vi "Camera_Trigger_Manual.vi"() -> ()   [LabVIEW 2022 SP3]
panel:
  in  "Trigger State":bool
  out "Cam 2":bool
  out "Cam 1":bool
  # "HW Trigger Control"
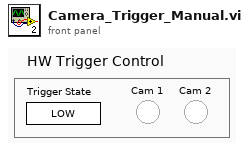
[diagram p1: front panel]
types:
  T1 = enum32{"Invalid", "Standard", "Closed", "Hidden", "Minimized", "Maximized"}
  T2 = enum32{"invalid app kind", "Development System", "Run Time System", "Student Edition", "Embedded LabVIEW", "Evaluation", "Custom"}
  T3 = typedef "Data.ctl" = cluster{"system":cluster{"info":cluster{"menuSelect":u16, "version":u16, "serial":string, "captureActive":bool, "captureBegin":bool, "emptyAndRefill":bool}, "userInfo":cluster{"operatorName":string, "date":timestamp}, "camera":cluster{"exposureTime":i32, "aperture":enum32{"Item 0", "Item 1", "Item 2", "Item 3"}, "framerate":i32, "framerateMax":i32, "legacyAttributes":bool}}, "connections":cluster{"arduino":cluster{"connection":refnum<visa-resource-name>, "status":bool, "openState":bool, "emptyStart":u32}, "pump":cluster{"connection":refnum<visa-resource-name>, "status":bool, "command":string, "dispenseSpeed":i32, "flushSize":i32}, "camera":cluster{"cam1":cluster{"connection":T4, "status":bool}, "cam2":cluster{"connection":T4, "status":bool}}}, "queue":cluster{"process":cluster{"cam1":refnum<queue>, "cam2":refnum<queue>, "queueSize":i32}, "save":cluster{"cam1":refnum<queue>, "cam2":refnum<queue>, "queueSize":i32}, "overloadThreshold":i32}, "imageProcess":cluster{"cam1":cluster{"preAllocation":cluster{"image":T5, "originalDisplay":T5, "originalRgb":T5, "binary":T5, "save":T5, "calibrationFull":T5, "calibrationDetect":T5}, "calibration":cluster{"pathFull":path, "pathDetect":path, "ROI":T6}}, "cam2":cluster{"preAllocation":cluster{"image":T5, "originalDisplay":T5, "originalRgb":T5, "binary":T5, "save":T5, "calibrationFull":T5, "calibrationDetect":T5}, "calibration":cluster{"pathFull":path, "pathDetect":path, "ROI":T6}}, "process":cluster{"planeExtract":T5, "planeSubtract":T5, "cropMask":T5}, "detection":cluster{"sampleTimeout":i32, "sizeThreshold":i32, "detectionRegionPct":dbl}}, "sampleData":cluster{"sampleId":string, "projectId":string, "voucherID":string, "speciesName":string, "collectionDate":timestamp, "sampleStation":string, "location":string, "lat":dbl, "lon":dbl, "determiner":string, "sex":string, "otherNotes":string}, "Session In":T4}
  T4 = typedef "IMAQdx.ctl" = refnum<k21>
  T5 = typedef "IMAQ Image.ctl" = refnum<image>
  T6 = typedef "IMAQ Rectangle" = cluster{"Left":i32, "Top":i32, "Right":i32, "Bottom":i32, "Rotation":dbl}
  T7 = cluster{"Core":cluster{"Current VI Reference":refnum<vi>, "Close Panel on Exit?":bool}, "value":T3}
  T8 = cluster{"Current VI Reference":refnum<vi>, "Close Panel on Exit?":bool}
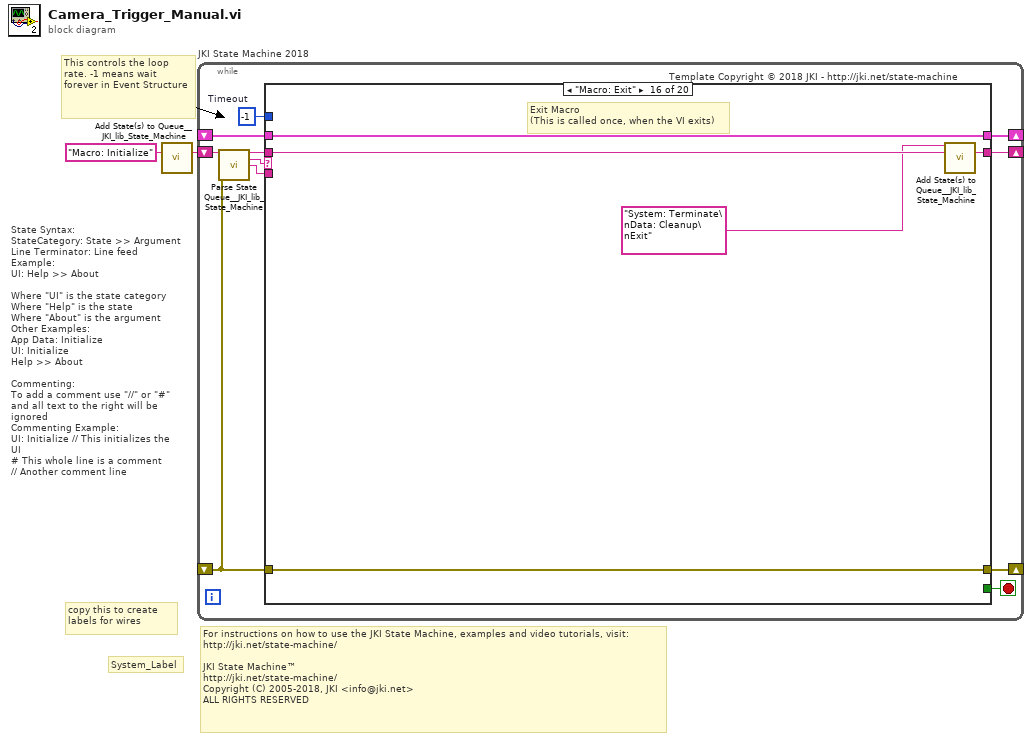
[diagram p0: block diagram]
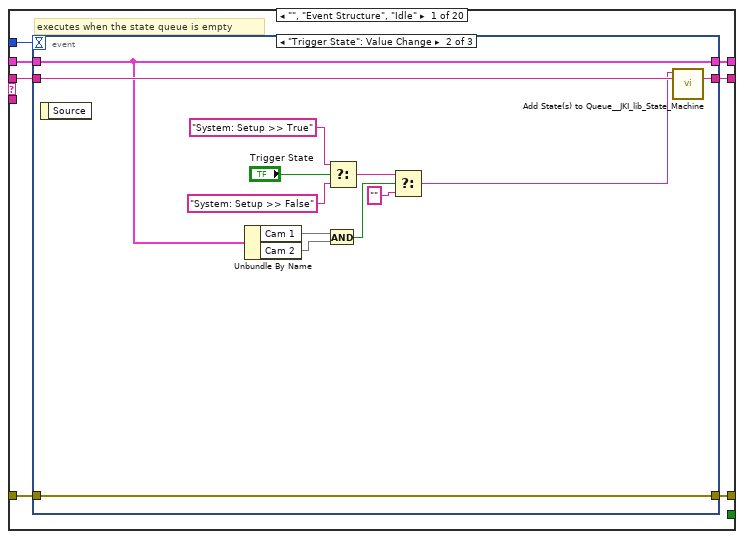
[diagram p2: hidden frame]
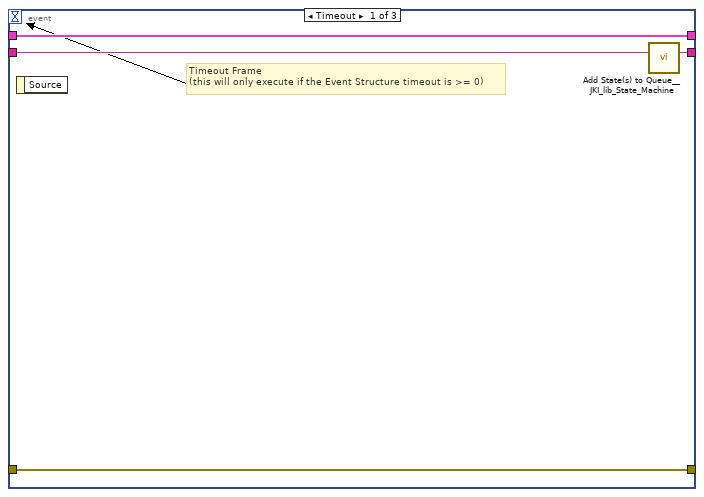
[diagram p3: hidden frame]
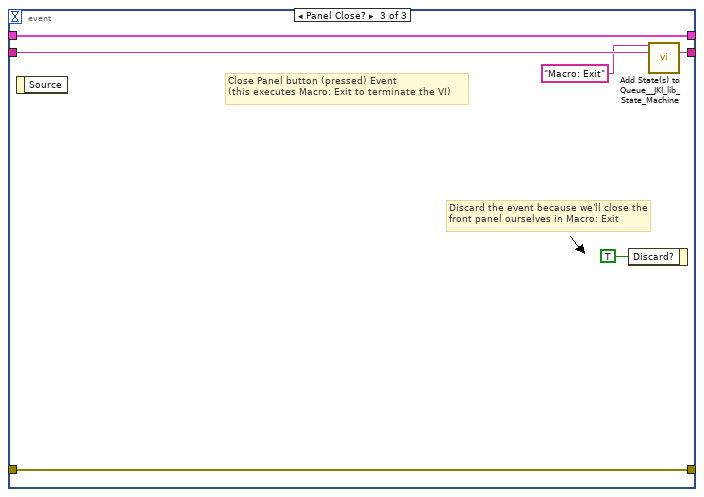
[diagram p4: hidden frame]
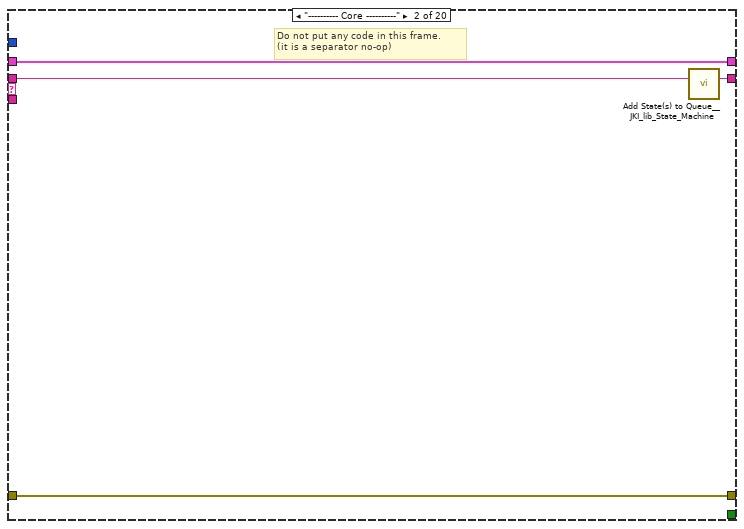
[diagram p5: hidden frame]
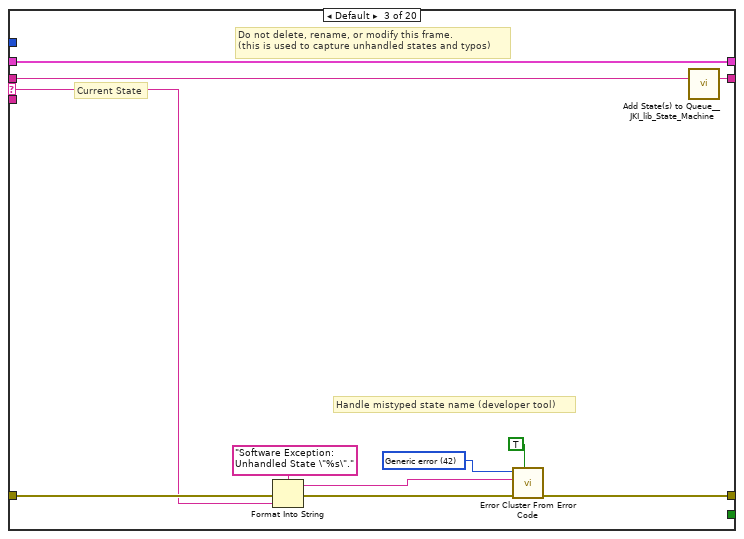
[diagram p6: hidden frame]
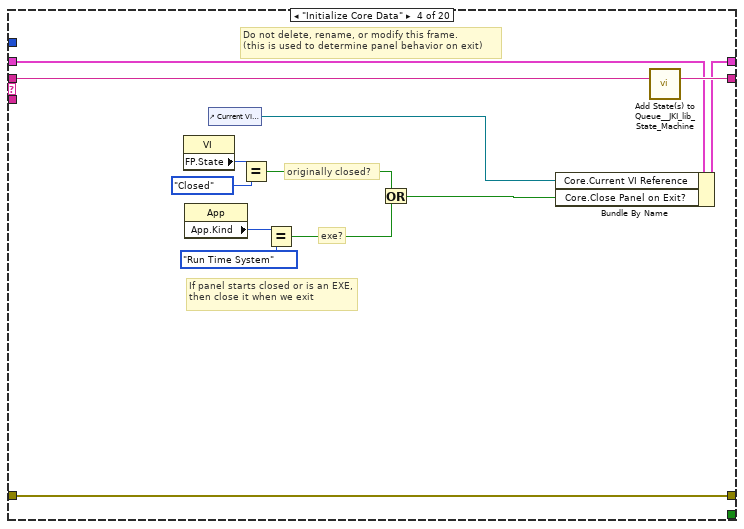
[diagram p7: hidden frame]
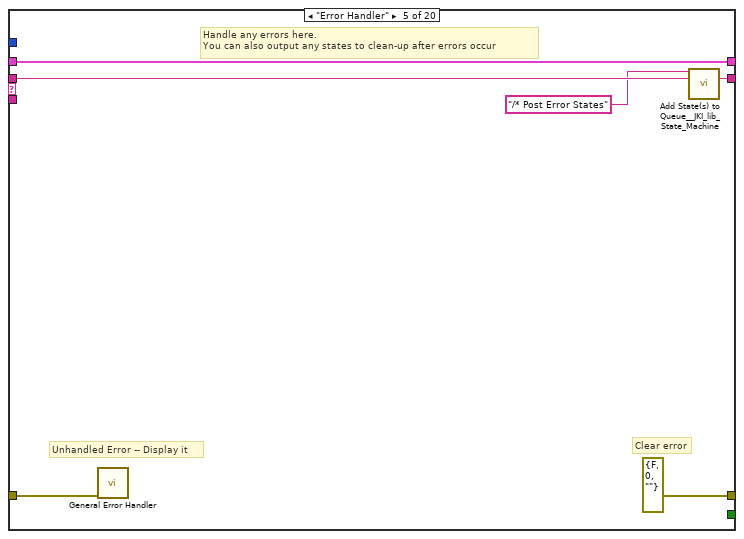
[diagram p8: hidden frame]
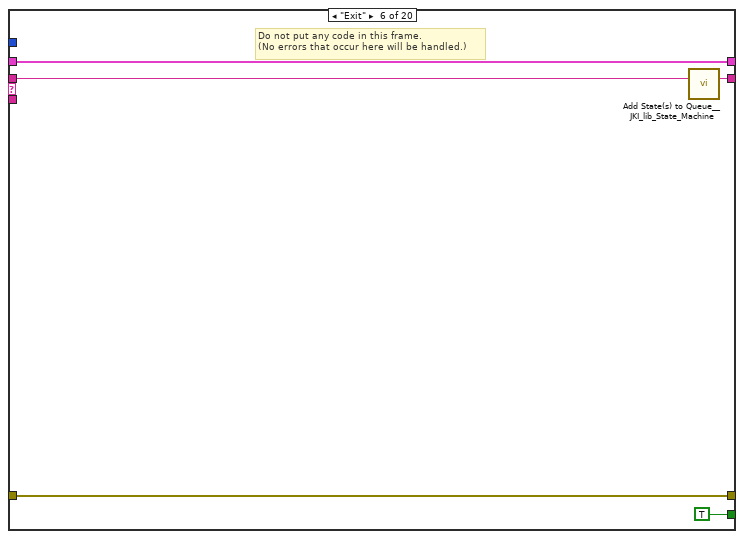
[diagram p9: hidden frame]
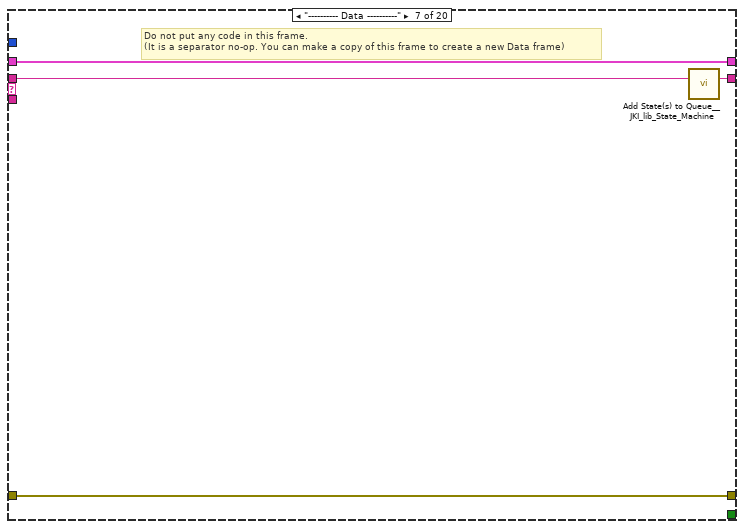
[diagram p10: hidden frame]
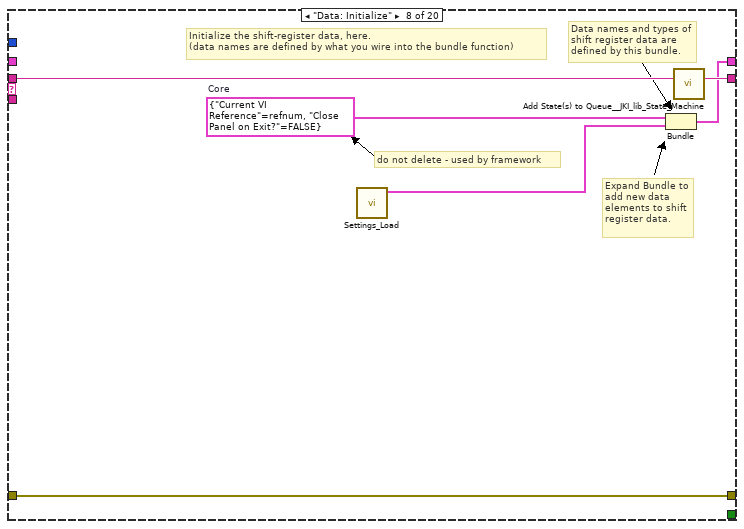
[diagram p11: hidden frame]
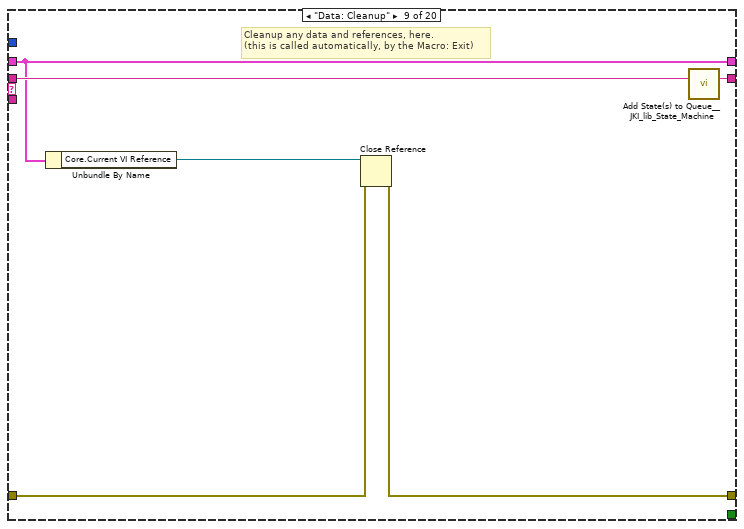
[diagram p12: hidden frame]
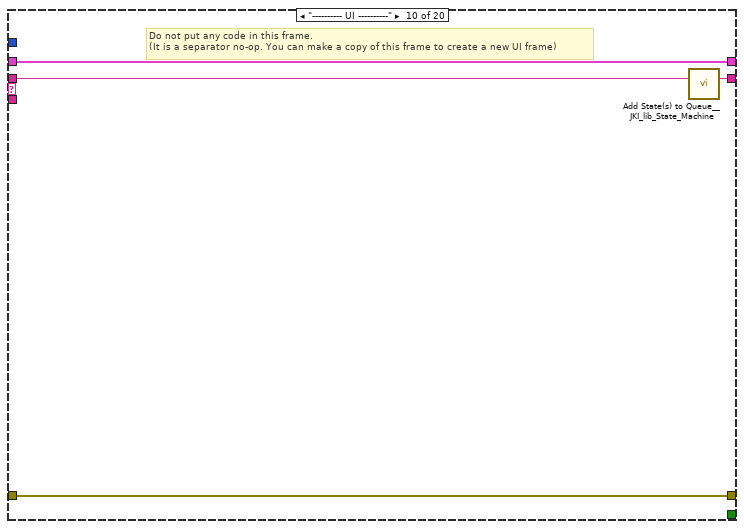
[diagram p13: hidden frame]
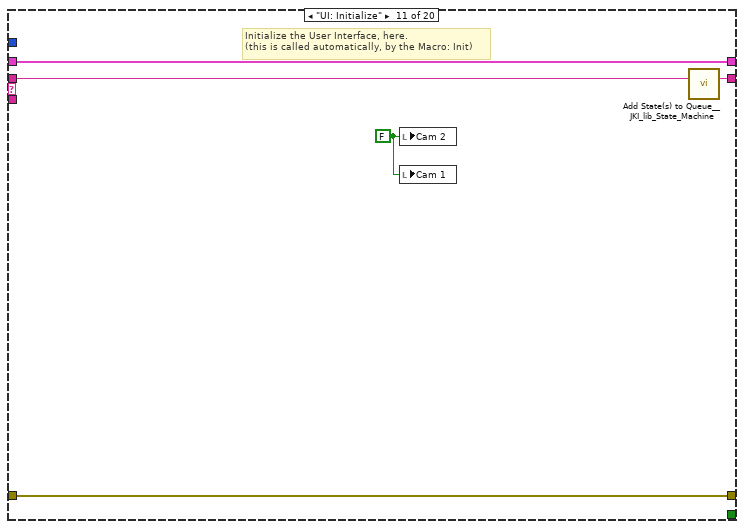
[diagram p14: hidden frame]
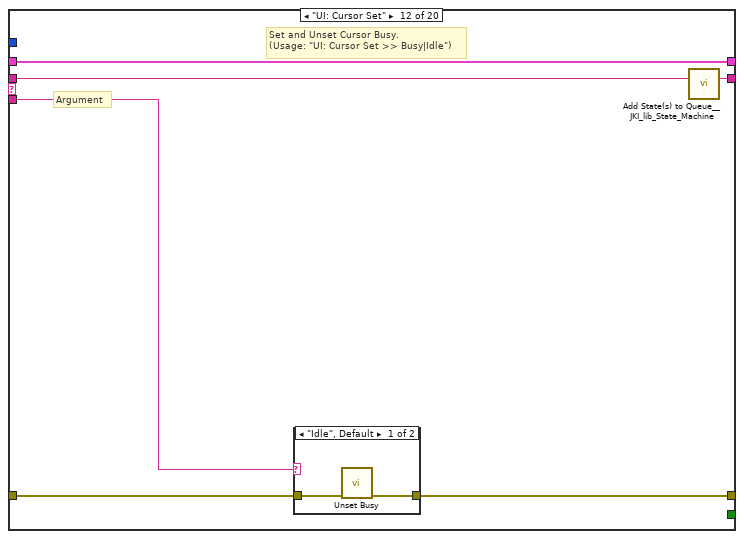
[diagram p15: hidden frame]
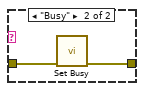
[diagram p16: hidden frame]
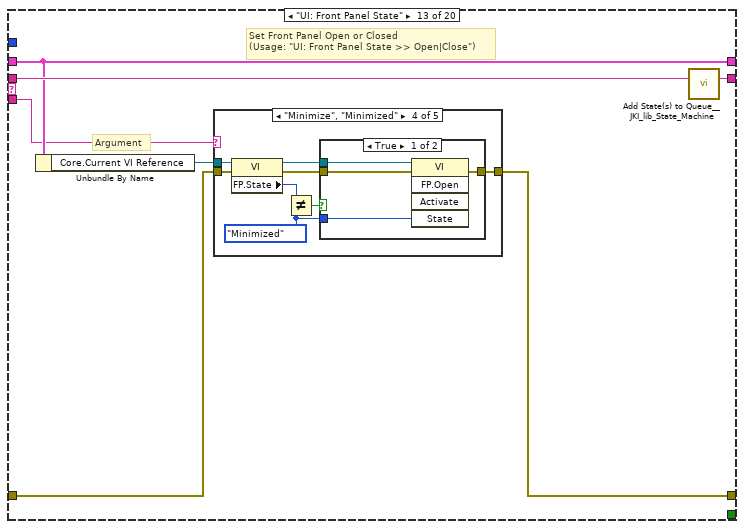
[diagram p17: hidden frame]
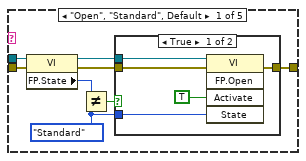
[diagram p18: hidden frame]
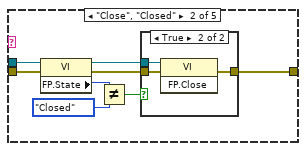
[diagram p20: hidden frame]
diagram:
  # "For instructions on how to use the JKI State Machine, examples and video tutorials, visit:\nhttp://jki.net/state-machine/\n\nJKI State Machine™\nhttp://jki.net/state-machine/\nCopyright (C) 2005-2018, JKI <info@jki.net>\nALL RIGHTS RESERVED"
  # "State Syntax:\nStateCategory: State >> Argument\nLine Terminator: Line feed\nExample:\nUI: Help >> About\n\nWhere \"UI\" is the state category\nWhere \"Help\" is the state\nWhere \"About\" is the argument\nOther Examples:\nApp Data: Initialize\nUI: Initialize\nHelp >> About\n\nCommenting:\nTo add a comment use \"//\" or \"#\" and all text to the right will be ignored\nCommenting Example:\nUI: Initialize // This initializes the UI\n# This whole line is a comment\n// Another comment line"
  # "copy this to create labels for wires"
  # "This controls the loop rate. -1 means wait forever in Event Structure"
  # "System_Label"
  n1 = call <vilib>:"Add State(s) to Queue__JKI_lib_State_Machine.vi"("State(s) in (\"\")"="Macro: Initialize") -> ("States Out"=w2:string)  [unwired: 14 in]
  n2 = while "JKI State Machine 2018" {
    shift-right: [w6] -> _
    shift-left: _ -> [w5]
    shift-right: [w9] -> _
    shift-left: _ -> [w3]
    shift-right: [w8] -> _
    shift-left: w2 -> [w10]
    stop <- w7 stop-if-true
    w4 = -1  # Timeout
    # "Template Copyright © 2018 JKI - http://jki.net/state-machine"
    n3 = call <vilib>:"Parse State Queue__JKI_lib_State_Machine.vi"("State Queue"=w10, "Error In (no error)"=w3) -> ("Remaining States"=w12:string, "Current State"=w13:string, "Arguments"=w11:string)  [unwired: 11 in]
    n4 = case shown="\"Macro: Exit\"" w13 {
      selector: w13 -> [_ _ w48 _ _ _ _ _ _ _ _ _ _ _ _ _ _ _ _ _]
      tunnel: w12 -> [w20 w47 w52 w71 w77 w82 w86 w92 w98 w102 w107 w113 w124 w193 w198 w203 w207 w218 w225 w233]
      tunnel: w11 -> [_ _ _ _ _ _ _ _ _ _ _ w108 w118 _ _ _ _ _ _ w228]
      tunnel: w5 -> [w18 w44 w50 w64 w74 w80 w83 _ w93 w99 w105 w111 w120 w190 w195 w200 w204 w213 w221 w231]
      tunnel: [w17 w45 w54 w68 errorcluster {"status"=FALSE, "code"=0, "source"=""} ("error out") w79 w84 w89 w94 w100 w104 w109 w121 w191 w196 w201 w205 w216 w223 w226] -> w9
      tunnel: w3 -> [w16 w45 w53 w68 w73 w79 w84 w89 w95 w100 w104 w110 w122 w191 w196 w201 w205 w216 w223 w230]
      tunnel: [w19 w46 w51 w70 w76 w81 w85 w91 w97 w101 w106 w112 w123 w192 w197 w202 w206 w217 w224 w232] -> w8
      tunnel: [_ _ _ _ _ TRUE _ _ _ _ _ _ _ _ _ _ _ _ _ _] -> w7
      tunnel: [w15 w44 w50 w69 w74 w80 w83 w90 w93 w99 w105 w111 w120 w190 w195 w200 w204 w211 w220 w231] -> w6
      tunnel: w4 -> [w14 _ _ _ _ _ _ _ _ _ _ _ _ _ _ _ _ _ _ _]
      frame "", "Event Structure", "Idle" {
        # "executes when the state queue is empty"
        n5 = event shown="[1] \"Trigger State\": Value Change" {
          selector: _ -> [_ _ _]
          dyn-events: _ -> [_ _ _]
          timeout: w14 -> [_ _ _]
          tunnel: w20 -> [w24 w37 w43]
          tunnel: [w23 w36 w42] -> w19
          tunnel: w18 -> [w21 w32 w40]
          tunnel: [w22 w35 w41] -> w17
          tunnel: w16 -> [w22 w35 w41]
          tunnel: [w21 w32 w40] -> w15
          event Timeout {
            # "Timeout Frame\n(this will only execute if the Event Structure timeout is >= 0)"
            n6 = event-data() -> ()  [unwired: 1 in, 1 out]
            n7 = call <vilib>:"Add State(s) to Queue__JKI_lib_State_Machine.vi"("State(s) in (\"\")"=w24) -> ("States Out"=w23:string)  [unwired: 14 in]
          }
          event "Trigger State": Value Change {
            n8 = event-data() -> ()  [unwired: 1 in, 1 out]
            n9 = Unbundle By Name(w32) -> ("Cam 1"=w30, "Cam 2"=w29)
            n10 = And(x=w30, y=w29) -> (x .and. y?=w28:bool)
            n11 = Select(t="System: Setup >> True" ("State(s) in Front (\"\")"), s="Trigger State", f="System: Setup >> False" ("State(s) in Front (\"\")")) -> (s? t:f=w27:string)
            n12 = Select(t=w27, s=w28, f="") -> (s? t:f=w25:string)
            n13 = call <vilib>:"Add State(s) to Queue__JKI_lib_State_Machine.vi"("State(s) in Front (\"\")"=w25, "State(s) in (\"\")"=w37) -> ("States Out"=w36:string)  [unwired: 13 in]
          }
          event Panel Close? {
            # "Discard the event because we'll close the front panel ourselves in Macro: Exit"
            # "Close Panel button (pressed) Event\n(this executes Macro: Exit to terminate the VI)"
            n14 = event-data() -> ()  [unwired: 1 in, 1 out]
            n15 = event-data("Discard?"=TRUE) -> ()  [unwired: 1 in, 1 out]
            n16 = call <vilib>:"Add State(s) to Queue__JKI_lib_State_Machine.vi"("State(s) in Front (\"\")"="Macro: Exit", "State(s) in (\"\")"=w43) -> ("States Out"=w42:string)  [unwired: 13 in]
          }
        }
      }
      frame "---------- Core ----------" {
        # "Do not put any code in this frame.\n(it is a separator no-op)"
        n17 = call <vilib>:"Add State(s) to Queue__JKI_lib_State_Machine.vi"("State(s) in (\"\")"=w47) -> ("States Out"=w46:string)  [unwired: 14 in]
      }
      frame Default {
        w57 = 42 items=["No error", "Argument error", "Memory is full", "Out of zone", "End of file", "File already open", "Generic file I/O error", "File not found", "File permission error", "Disk is full", "Duplicate path", "Too many files open", "System feature not enabled", "Resource file not found", "Cannot add resource", "Resource not found", "Image not found", "Image memory error", "Pen does not exist", "Config type invalid", "Config token not found", "Config parse error", "Config memory error", "Bad external code format", "Bad external code offset", "External code not present", "Null window", "Destroy window error", "Null menu", "Print aborted", "Bad print record", "Print driver error", "Windows error during printing", "Memory error during printing", "Print dialog error", "Generic print error", "Invalid device refnum", "Device not found", "Device parameter error", "Device unit error", "Cannot open device", "Device call aborted", "Generic error", "Cancelled by user", "Object ID too low", "Object ID too high", "Object not in heap", "Unknown heap", "Unknown object (invalid DefProc)", "Unknown object (DefProc not in table)", "Message out of range", "Invalid (null) method", "Unknown message", "Manager call not supported", "Bad address", "Network operation in progress", "Network operation timed out", "Connection is busy", "Network attribute not supported", "Network error", "Address in use", "System out of memory", "Connection aborted", "Connection refused", "Not connected", "Already connected", "Connection closed", "Initialization error (interapplication manager)", "Bad occurrence", "Wait on unbound occurrence handler", "Occurrence queue overflow", "Datalog type conflict", "Unused", "Unrecognized type (interapplication manager)", "Memory corrupt", "Failed to make temporary DLL", "Old CIN version", "Drag socket not found", "Failed to load drop-object", "Failed to register OLE object", "Failed to release OLE object", "Format specifier type mismatch", "Unknown format specifier", "Too few format specifiers", "Too many format specifiers", "Scan failed", "Newer CIN version", "Error converting to variant", "Runtime menu error", "Password tampered", "Variant attribute not found", "Incompatible variant data type", "Event data is not available", "Event Store is not present", "Occurrence is not found", "Event Queue is not created", "Event info is not available", "Refnum passed is NULL", "Error retrieving Class GUID", "Error retrieving CoClass GUID", "Error retrieving TypeLib GUID.", "Bad built application magic bytes.", "Specific driver is different from the specific driver associated with the Logical Name.", "There is no session opened to the class driver.", "Max Error", "MAX - Error with config objects", "MAX - Error loading configuration", "MAX - Group not supported"]
        # "Current State"
        # "Do not delete, rename, or modify this frame.\n(this is used to capture unhandled states and typos)"
        # "Handle mistyped state name (developer tool)"
        n18 = Format Into String(format string="Software Exception: Unhandled State \"%s\"." ("message"), error in=w53, w48) -> (resulting string=w56:string, error out=w55:errorcluster)  [unwired: 1 in]
        n19 = call <vilib>:"Error Cluster From Error Code.vi"("show call chain? (False)"=TRUE, "error in (no error)"=w55, "error message (\"\")"=w56, "error code (0)"=w57) -> ("error out"=w54:errorcluster)  [unwired: 5 in]
        n20 = call <vilib>:"Add State(s) to Queue__JKI_lib_State_Machine.vi"("State(s) in (\"\")"=w52) -> ("States Out"=w51:string)  [unwired: 14 in]
      }
      frame "Initialize Core Data" {
        # "Do not delete, rename, or modify this frame.\n(this is used to determine panel behavior on exit)"
        # "originally closed?"
        # "exe?"
        # "If panel starts closed or is an EXE, then close it when we exit"
        n21 = property class="VI"() -> ("FP.State"=w61:T1)  [unwired: 2 in, 2 out]
        n22 = property class="App"() -> ("App.Kind"=w67:T2)  [unwired: 2 in, 2 out]
        n23 = control-ref of="Current VI Reference"() -> (w62:refnum<vi>)
        n24 = Equal?(x=w61, y=T1."Closed" ("Front Panel Window:State")) -> (x = y?=w59:bool)
        n25 = Equal?(x=w67, y=T2."Run Time System" ("Application:Kind")) -> (x = y?=w65:bool)
        n26 = Or(x=w59, y=w65) -> (x .or. y?=w63:bool)
        n27 = Bundle By Name(cluster=w64, "Core.Current VI Reference"=w62, "Core.Close Panel on Exit?"=w63) -> (w69:T7)
        n28 = call <vilib>:"Add State(s) to Queue__JKI_lib_State_Machine.vi"("State(s) in (\"\")"=w71) -> ("States Out"=w70:string)  [unwired: 14 in]
      }
      frame "Error Handler" {
        # "Unhandled Error -- Display it"
        # "Handle any errors here.\nYou can also output any states to clean-up after errors occur"
        # "Clear error"
        n29 = call <vilib>:"General Error Handler.vi"("error in (no error)"=w73) -> ()  [unwired: 10 in, 5 out]
        n30 = call <vilib>:"Add State(s) to Queue__JKI_lib_State_Machine.vi"("State(s) in Front (\"\")"="/* Post Error States", "State(s) in (\"\")"=w77) -> ("States Out"=w76:string)  [unwired: 13 in]
      }
      frame "Exit" {
        # "Do not put any code in this frame.\n(No errors that occur here will be handled.)"
        n31 = call <vilib>:"Add State(s) to Queue__JKI_lib_State_Machine.vi"("State(s) in (\"\")"=w82) -> ("States Out"=w81:string)  [unwired: 14 in]
      }
      frame "---------- Data ----------" {
        # "Do not put any code in this frame.\n(It is a separator no-op. You can make a copy of this frame to create a new Data frame)"
        n32 = call <vilib>:"Add State(s) to Queue__JKI_lib_State_Machine.vi"("State(s) in (\"\")"=w86) -> ("States Out"=w85:string)  [unwired: 14 in]
      }
      frame "Data: Initialize" {
        w88 = T8 {"Current VI Reference"=refnum, "Close Panel on Exit?"=FALSE}  # Core
        # "do not delete - used by framework"
        # "Expand Bundle to add new data elements to shift register data."
        # "Data names and types of shift register data are defined by this bundle."
        # "Initialize the shift-register data, here.\n(data names are defined by what you wire into the bundle function)"
        n33 = call "Settings_Load.vi"() -> ("value"=w87:T3)  [unwired: 10 in, 1 out]
        n34 = Bundle("Core"=w88, "value"=w87) -> (w90:T7)  [unwired: 1 in]
        n35 = call <vilib>:"Add State(s) to Queue__JKI_lib_State_Machine.vi"("State(s) in (\"\")"=w92) -> ("States Out"=w91:string)  [unwired: 14 in]
      }
      frame "Data: Cleanup" {
        # "Cleanup any data and references, here.\n(this is called automatically, by the Macro: Exit)"
        n36 = Unbundle By Name(w93) -> ("Core.Current VI Reference"=w96:refnum<vi>)
        n37 = Close Reference(reference=w96, error in (no error)=w95) -> (error out=w94:errorcluster)
        n38 = call <vilib>:"Add State(s) to Queue__JKI_lib_State_Machine.vi"("State(s) in (\"\")"=w98) -> ("States Out"=w97:string)  [unwired: 14 in]
      }
      frame "---------- UI ----------" {
        # "Do not put any code in this frame.\n(It is a separator no-op. You can make a copy of this frame to create a new UI frame)"
        n39 = call <vilib>:"Add State(s) to Queue__JKI_lib_State_Machine.vi"("State(s) in (\"\")"=w102) -> ("States Out"=w101:string)  [unwired: 14 in]
      }
      frame "UI: Initialize" {
        w103 = FALSE ("Cam 2")
        # "Initialize the User Interface, here.\n(this is called automatically, by the Macro: Init)"
        n40 = local write "Cam 2"(w103) -> ()
        n41 = local write "Cam 1"(w103) -> ()
        n42 = call <vilib>:"Add State(s) to Queue__JKI_lib_State_Machine.vi"("State(s) in (\"\")"=w107) -> ("States Out"=w106:string)  [unwired: 14 in]
      }
      frame "UI: Cursor Set" {
        # "Argument"
        # "Set and Unset Cursor Busy.\n(Usage: \"UI: Cursor Set >> Busy|Idle\")"
        n43 = case shown="\"Idle\", Default" w108 {
          tunnel: w110 -> [w115 w117]
          tunnel: [w114 w116] -> w109
          frame "Idle", Default {
            n44 = call <vilib>:"Unset Busy.vi"("error in (no error)"=w115) -> ("error out"=w114:errorcluster)  [unwired: 10 in]
          }
          frame "Busy" {
            n45 = call <vilib>:"Set Busy.vi"("error in (no error)"=w117) -> ("error out"=w116:errorcluster)  [unwired: 9 in, 1 out]
          }
        }
        n46 = call <vilib>:"Add State(s) to Queue__JKI_lib_State_Machine.vi"("State(s) in (\"\")"=w113) -> ("States Out"=w112:string)  [unwired: 14 in]
      }
      frame "UI: Front Panel State" {
        # "Argument"
        # "Set Front Panel Open or Closed\n(Usage: \"UI: Front Panel State >> Open|Close\")"
        n47 = Unbundle By Name(w120) -> ("Core.Current VI Reference"=w119:refnum<vi>)
        n48 = case shown="\"Minimize\", \"Minimized\"" w118 {
          tunnel: w122 -> [w130 w145 w156 w169 w182]
          tunnel: [w132 w146 w158 w171 w184] -> w121
          tunnel: w119 -> [w131 w143 w157 w170 w183]
          frame "Open", "Standard", Default {
            w125 = T1."Standard" ("State")
            n49 = property class="VI"(reference=w131, error in=w130) -> (reference out=w128:refnum<vi>, error out=w129:errorcluster, "FP.State"=w127:T1)
            n50 = Not Equal?(x=w127, y=w125) -> (x != y?=w126:bool)
            n51 = case shown="True" w126 {
              tunnel: [w136 w138] -> w132
              tunnel: w129 -> [w135 w138]
              tunnel: w128 -> [w134 _]
              tunnel: w125 -> [w133 _]
              frame True {
                n52 = invoke class="VI" method="FP.Open"(reference=w134, error in=w135, "Activate"=TRUE, "State"=w133) -> (error out=w136:errorcluster)  [unwired: 1 in, 4 out]
              }
              frame False {
              }
            }
          }
          frame "Close", "Closed" {
            n53 = property class="VI"(reference=w143, error in=w145) -> (reference out=w142:refnum<vi>, error out=w144:errorcluster, "FP.State"=w140:T1)
            n54 = Not Equal?(x=w140, y=T1."Closed" ("Front Panel Window:State")) -> (x != y?=w139:bool)
            n55 = case shown="True" w139 {
              tunnel: [w147 w150] -> w146
              tunnel: w144 -> [w147 w149]
              tunnel: w142 -> [_ w148]
              frame False {
              }
              frame True {
                n56 = invoke class="VI" method="FP.Close"(reference=w148, error in=w149) -> (error out=w150:errorcluster)  [unwired: 1 in, 2 out]
              }
            }
          }
          frame "Hidden", "Hide" {
            w151 = T1."Hidden" ("State")
            n57 = property class="VI"(reference=w157, error in=w156) -> (reference out=w154:refnum<vi>, error out=w155:errorcluster, "FP.State"=w153:T1)
            n58 = Not Equal?(x=w153, y=w151) -> (x != y?=w152:bool)
            n59 = case shown="True" w152 {
              tunnel: [w162 w163] -> w158
              tunnel: w155 -> [w161 w163]
              tunnel: w154 -> [w160 _]
              tunnel: w151 -> [w159 _]
              frame True {
                n60 = invoke class="VI" method="FP.Open"(reference=w160, error in=w161, "State"=w159) -> (error out=w162:errorcluster)  [unwired: 2 in, 4 out]
              }
              frame False {
              }
            }
          }
          frame "Minimize", "Minimized" {
            w164 = T1."Minimized" ("State")
            n61 = property class="VI"(reference=w170, error in=w169) -> (reference out=w167:refnum<vi>, error out=w168:errorcluster, "FP.State"=w166:T1)
            n62 = Not Equal?(x=w166, y=w164) -> (x != y?=w165:bool)
            n63 = case shown="True" w165 {
              tunnel: [w175 w176] -> w171
              tunnel: w168 -> [w174 w176]
              tunnel: w167 -> [w173 _]
              tunnel: w164 -> [w172 _]
              frame True {
                n64 = invoke class="VI" method="FP.Open"(reference=w173, error in=w174, "State"=w172) -> (error out=w175:errorcluster)  [unwired: 2 in, 4 out]
              }
              frame False {
              }
            }
          }
          frame "Maximize", "Maximized" {
            w177 = T1."Maximized" ("State")
            n65 = property class="VI"(reference=w183, error in=w182) -> (reference out=w180:refnum<vi>, error out=w181:errorcluster, "FP.State"=w179:T1)
            n66 = Not Equal?(x=w179, y=w177) -> (x != y?=w178:bool)
            n67 = case shown="True" w178 {
              tunnel: [w188 w189] -> w184
              tunnel: w181 -> [w187 w189]
              tunnel: w180 -> [w186 _]
              tunnel: w177 -> [w185 _]
              frame True {
                n68 = invoke class="VI" method="FP.Open"(reference=w186, error in=w187, "State"=w185) -> (error out=w188:errorcluster)  [unwired: 2 in, 4 out]
              }
              frame False {
              }
            }
          }
        }
        n69 = call <vilib>:"Add State(s) to Queue__JKI_lib_State_Machine.vi"("State(s) in (\"\")"=w124) -> ("States Out"=w123:string)  [unwired: 14 in]
      }
      frame "---------- Macro ----------" {
        # "Do not put any code in this frame.\n(It is a separator no-op. You can make a copy of this frame to create a new Macro frame)"
        n70 = call <vilib>:"Add State(s) to Queue__JKI_lib_State_Machine.vi"("State(s) in (\"\")"=w193) -> ("States Out"=w192:string)  [unwired: 14 in]
      }
      frame "Macro: Initialize" {
        w194 = "Data: Initialize\nInitialize Core Data\nUI: Initialize\nSystem: Connect\nUI: Front Panel State >> Open"  # Data: Initialize Initialize Core Data UI: Initialize System: Connect UI: Front Panel State >> Open
        # "Initialization Macro\n(This is called once, when the VI starts)"
        n71 = call <vilib>:"Add State(s) to Queue__JKI_lib_State_Machine.vi"("State(s) in Front (\"\")"=w194, "State(s) in (\"\")"=w198) -> ("States Out"=w197:string)  [unwired: 13 in]
      }
      frame "Macro: Exit" {
        # "Exit Macro\n(This is called once, when the VI exits)"
        n72 = call <vilib>:"Add State(s) to Queue__JKI_lib_State_Machine.vi"("State(s) in Front (\"\")"="System: Terminate\nData: Cleanup\nExit", "State(s) in (\"\")"=w203) -> ("States Out"=w202:string)  [unwired: 13 in]
      }
      frame "---------- System ----------" {
        # "Template Separator\n(You can make a copy of, or modify, this frame)"
        n73 = call <vilib>:"Add State(s) to Queue__JKI_lib_State_Machine.vi"("State(s) in (\"\")"=w207) -> ("States Out"=w206:string)  [unwired: 14 in]
      }
      frame "System: Connect" {
        # "Your code here.\n(You can make a copy of, or modify, this frame)"
        n74 = Unbundle By Name(w213) -> ("value"=w214:T3)
        n75 = call "Terminate_Connection.vi"("Data"=w214) -> ("error out"=w210:errorcluster, "Data out"=w215:T3)  [unwired: 9 in]
        n76 = call "Connections.vi"("input cluster"=w215, "error in"=w210) -> ("output cluster"=w212:T3, "Camear 1"=→"Cam 1":bool, "Camera 2"=→"Cam 2":bool)  [unwired: 8 in, 3 out]
        n77 = Bundle By Name(cluster=w213, "value"=w212) -> (w211:T7)
        n78 = call <vilib>:"Add State(s) to Queue__JKI_lib_State_Machine.vi"("State(s) in (\"\")"=w218) -> ("States Out"=w217:string)  [unwired: 14 in]
      }
      frame "System: Terminate" {
        # "Your code here.\n(You can make a copy of, or modify, this frame)"
        n79 = Unbundle By Name(w221) -> ("value"=w222:T3)
        n80 = call "Terminate_Connection.vi"("Data"=w222) -> ("Data out"=w219:T3)  [unwired: 9 in, 1 out]
        n81 = Bundle By Name(cluster=w221, "value"=w219) -> (w220:T7)
        n82 = call <vilib>:"Add State(s) to Queue__JKI_lib_State_Machine.vi"("State(s) in (\"\")"=w225) -> ("States Out"=w224:string)  [unwired: 14 in]
      }
      frame "System: Setup" {
        # "Your code here.\n(You can make a copy of, or modify, this frame)"
        n83 = case shown="\"False\", Default" w228 {
          tunnel: [FALSE TRUE] -> w227
          frame "False", Default {
          }
          frame "True" {
          }
        }
        n84 = Unbundle By Name(w231) -> ("value"=w229:T3)
        n85 = call "Camera_Config_Manual.vi"("error in"=w230, "Trigger state"=w227, "input cluster"=w229) -> ("error out"=w226:errorcluster)  [unwired: 8 in]
        n86 = call <vilib>:"Add State(s) to Queue__JKI_lib_State_Machine.vi"("State(s) in (\"\")"=w233) -> ("States Out"=w232:string)  [unwired: 14 in]
      }
    }
  }
